vi "GetImagetoIMAQ.vi"(8 "error in (no error)":errorcluster, 10 "Image Src":T1, 11 "Image Data":T2) -> (0 "error out":errorcluster, 3 "Image Out":T1)   [LabVIEW 2017]
uses:
  <vilib>/picture/picture.llb/imagedata.ctl
  <vilib>/vision/Image Controls.llb/IMAQ Image.ctl
  <vilib>/vision/NI_Vision_Development_Module.lvlib
panel:
  out "min value":u32
  out "max value":u32
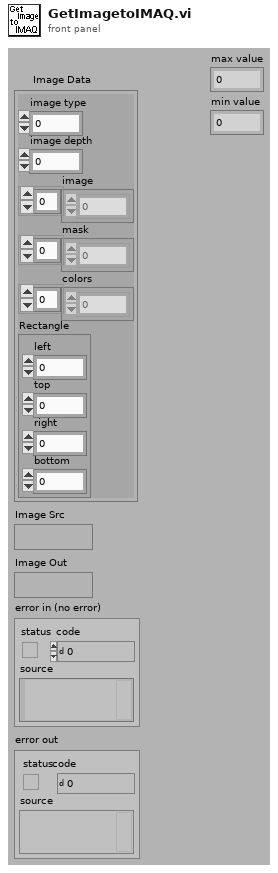
[diagram p1: front panel]
types:
  T1 = typedef "IMAQ Image.ctl" = refnum<image>
  T2 = typedef "imagedata.ctl" = cluster{"image type":i32, "image depth":i32, "image":u8[], "mask":u8[], "colors":u32[], "Rectangle":cluster{"left":i16, "top":i16, "right":i16, "bottom":i16}}
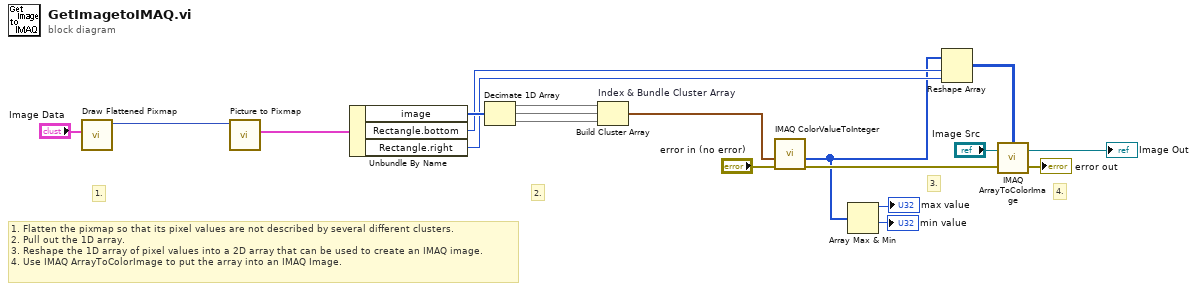
[diagram p0: block diagram]
diagram:
  # "1. Flatten the pixmap so that its pixel values are not described by several different clusters.\n2. Pull out the 1D array.\n3. Reshape the 1D array of pixel values into a 2D array that can be used to create an IMAQ image.\n4. Use IMAQ ArrayToColorImage to put the array into an IMAQ Image."
  # "4."
  # "3."
  # "2."
  # "1."
  n1 = call <vilib>:"Draw Flattened Pixmap.vi"("image data"="Image Data") -> ("new picture"=w19:picture)  [unwired: 8 in]
  n2 = call <vilib>:"Picture to Pixmap.vi"("picture"=w19) -> ("image data"=w17:T2)  [unwired: 9 in, 1 out]
  n3 = Unbundle By Name "Unbundle By Name"(w17) -> ("image"=w16:u8[], "Rectangle.bottom"=w11:i16, "Rectangle.right"=w10:i16)
  n4 = Decimate 1D Array "Decimate 1D Array"(w16) -> (w15:u8[], w14:u8[], w13:u8[])
  n5 = Build Cluster Array "Index & Bundle Cluster Array"(w15, w14, w13) -> (w12:cluster{u8, u8, u8}[])
  n6 = call "IMAQ ColorValueToInteger"("error in (no error)"="error in (no error)", "1D Color value array"=w12) -> ("1D U32 array"=w4:u32[], "error out"=w6:errorcluster)  [unwired: 3 in, 2 out]
  n7 = Array Max & Min(array=w4) -> (max value=→"max value":u32, min value=→"min value":u32)  [unwired: 2 out]
  n8 = Reshape Array(w4, w11, w10) -> (w1:u32[][])
  n9 = call "IMAQ ArrayToColorImage"("Image Pixels (U32)"=w1, "Image"="Image Src", "error in (no error)"=w6) -> ("Image Out"=→"Image Out":T1, "error out"=→"error out":errorcluster)  [unwired: 2 in]
